vi "2-4 Deocder_Pramith.vi"() -> ()   [LabVIEW 2012]
panel:
  in  "stop":bool
  out "Y3":bool
  out "Y2":bool
  out "Y1":bool
  out "Y0":bool
  in  "Input (0,1)":bool
  in  "Input (0,1)":bool
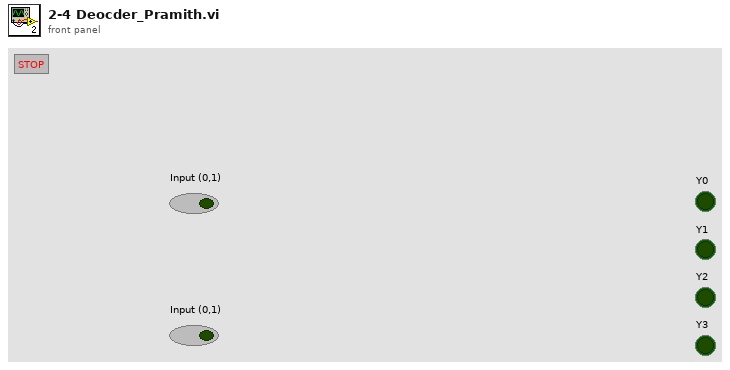
[diagram p1: front panel]
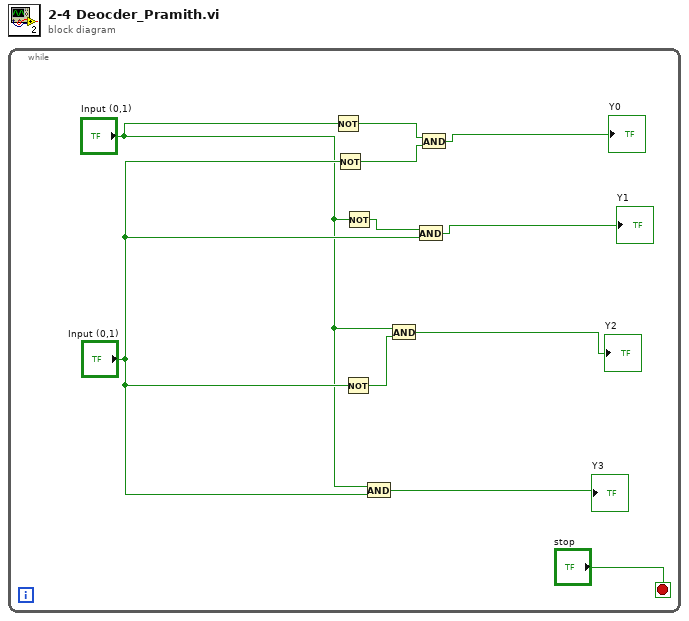
[diagram p0: block diagram]
diagram:
  n1 = while {
    stop <- "stop" stop-if-true
    n2 = Not(x="Input (0,1)") -> (.not. x?=w11:bool)
    n3 = Not(x="Input (0,1)") -> (.not. x?=w10:bool)
    n4 = Not(x="Input (0,1)") -> (.not. x?=w6:bool)
    n5 = Not(x="Input (0,1)") -> (.not. x?=w8:bool)
    n6 = And(x="Input (0,1)", y="Input (0,1)") -> (x .and. y?=→"Y3":bool)
    n7 = And(x="Input (0,1)", y=w6) -> (x .and. y?=→"Y2":bool)
    n8 = And(x=w8, y="Input (0,1)") -> (x .and. y?=→"Y1":bool)
    n9 = And(x=w11, y=w10) -> (x .and. y?=→"Y0":bool)
  }
